vi "orderbook.test.vi"() -> ()   [LabVIEW 2020]
uses:
  orderbook.command.type.ctl
  orderbook.variables.ctl
  application/orderbook.entry.ctl
  application/orderbook.result.type.ctl
  orderbook.state.ctl
  orderbook.memory.states.ctl
  <vilib>/Platform/TimedLoop/XDataNode/timing_clust.ctl
  <vilib>/Platform/TimedLoop/XDataNode/nitl_modes.ctl
  <vilib>/Platform/TimedLoop/XDataNode/wakeup.ctl
  orderbook.command.ctl
  <vilib>/rvi/Emulation/niFpgaSctlEmulationGetInTimedLoop.vi
  <vilib>/rvi/Emulation/niFpgaEmulationReportErrorSimple.vi
  <vilib>/rvi/Emulation/niFpgaGetClockAttributes.vi
  <vilib>/rvi/Emulation/niFpgaCriticalErrorInLSC.vi
  <vilib>/rvi/interface/RandomDataEmulation/nirviRandomDataMultiElementFPGAFIFO.vi
  <instcachedir>/0/nirviRandomDataMultiElementFPGAFIFO_3E9965BA1FAD4E7B8DABA31768A09B1F.lvgen/nirviRandomDataMultiElementFPGAFIFO_3E9965BA1FAD4E7B8DABA31768A09B1F_002.vi
  <vilib>/rvi/interface/RandomDataEmulation/niFpgaRandomDataHandleErrors.vi
  <vilib>/rvi/DataTransferAndStorage/Container/Common/niFpgaContainerExecOnDevCompGetState.vi
  <vilib>/rvi/Emulation/niFpgaEmulationIsFPGAContextNoSignature.vi
  <vilib>/rvi/errors/niFpgaSetErrorForExecOnDevCompSimple.vi
  <vilib>/rvi/eio/common/nirviEmuReportErrorAndStop.vi
  <vilib>/rvi/DataTransferAndStorage/Container/Common/niFpgaContainerGetUniqueNameForEmu.vi
  <vilib>/rvi/FIFO/Fifo_Resource/nirvififoEmulationSetSize.vi
  <vilib>/rvi/FIFO/Fifo_Resource/nirviFifoEmulationQueueMgr.vi
  <instcachedir>/0/nirviFifoEmulationQueueMgr_E5CAEC123FF24DC58D834DCA3CDAA9B5.lvgen/nirviFifoEmulationQueueMgr_E5CAEC123FF24DC58D834DCA3CDAA9B5_018.vi
  <vilib>/rvi/FIFO/Fifo_Resource/nirvififoEmulationDetermineInputValidOut.vi
  <vilib>/rvi/FIFO/Fifo_Resource/nirvififoEmulationCreateLock.vi
  <vilib>/rvi/Emulation/niFpgaProcessEmulError.vi
  <vilib>/rvi/FIFO/Fifo_Resource/nirvififoEmulationObtainLock.vi
  <vilib>/rvi/FIFO/Fifo_Resource/nirvififoEmulationReleaseLock.vi
  <vilib>/rvi/occurrence/nirviWaitOnOccurrenceBase.vi
  <vilib>/rvi/errors/nirviReportUnexpectedCaseInternalError.vi
  <vilib>/rvi/errors/nirviReportUnexpectedCaseInternalError (U32).vi
  <vilib>/Utility/error.llb/Clear Errors.vi
  <instcachedir>/0/nirviFifoEmulationQueueMgr_E5CAEC123FF24DC58D834DCA3CDAA9B5.lvgen/nirviFifoEmulationQueueMgr_E5CAEC123FF24DC58D834DCA3CDAA9B5_017.vi
  <vilib>/Platform/TimedLoop/XDataNode/XDataNode.xnode
  <vilib>/rvi/DataTransferAndStorage/Container/XNode/niFpgaContainer.xnode
  <vilib>/rvi/interface/RandomDataEmulation/nirviRandomDataFpgaMultiElementTemplate.vi
  <vilib>/rvi/FIFO/Fifo_Resource/niFpgaFifoEmulationRefIn.vi
  <vilib>/Platform/TimedLoop/XDataNode/XDNodeRunTimeDep.lvlib
panel:
  out "OrderBook.Variables":T1={"Write.Request"=FALSE, "Read.Request"=FALSE, "Read.Address"=0, "Read.OrderBook.Entry"={"OrderBook Result"=enum."Result.Found", "Side (U8)"=0, "Order Id (U64)"=0, "Quantity (U32)"=0, "Symbol (U64)"=0, "Price (U64)"=0, "Other Metric (U32)"=0, "Other Metric 2 (U32)"=0}, "Number.of.Entries"=0, "OrderBook.State"=enum."Reset", "Ready.For.OrderBook.Command"=FALSE, "Memory.State"=enum."Write", "Move"=FALSE, "Read.Valid"=FALSE, "Write.Address"=0, "Write.OrderBook.Entry"={"OrderBook Result"=enum."Result.Found", "Side (U8)"=0, "Order Id (U64)"=0, "Quantity (U32)"=0, "Symbol (U64)"=0, "Price (U64)"=0, "Other Metric (U32)"=0, "Other Metric 2 (U32)"=0}, "OrderBook.Result.Valid"=FALSE, "AddOrder.Count"=0, "Query.Count"=0, "Reset.Count"=0, "Wait.Count"=0}
  in  "Reset":bool
  in  "OrderBook Command":T6
  in  "Cancelled Quantity (U32)":u32
  in  "Executed Quantity (U32)":u32
  in  "Price (U64)":u64
  in  "Symbol (U64)":u64
  in  "Quantity (U32)":u32
  in  "Order Id (U64)":u64
  in  "Side (U8)":u8
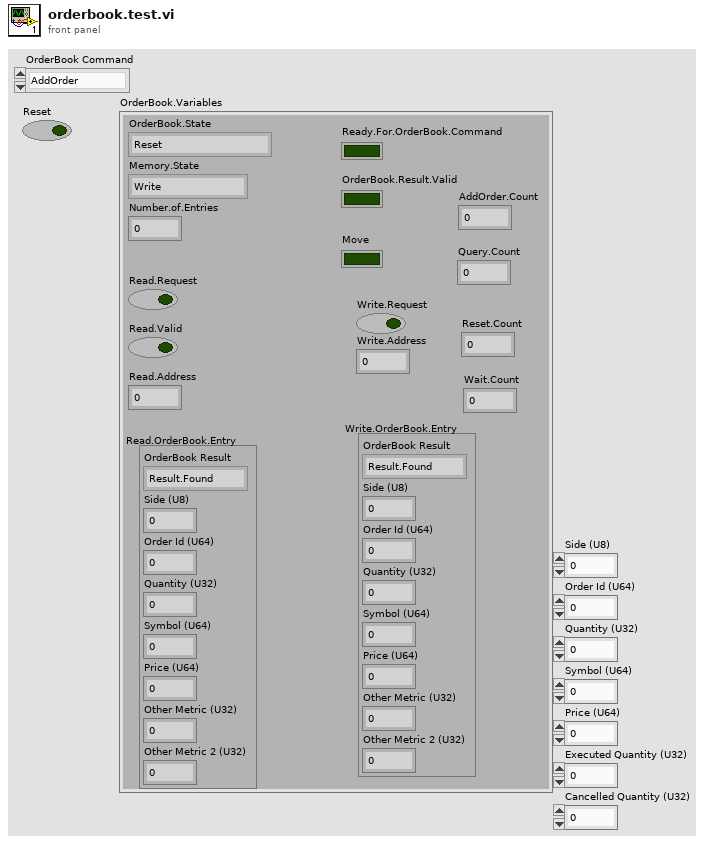
[diagram p1: front panel]
types:
  T1 = typedef "orderbook.variables.ctl" = cluster{"Write.Request":bool, "Read.Request":bool, "Read.Address":u32, "Read.OrderBook.Entry":T2, "Number.of.Entries":u32, "OrderBook.State":T4, "Ready.For.OrderBook.Command":bool, "Memory.State":T5, "Move":bool, "Read.Valid":bool, "Write.Address":u32, "Write.OrderBook.Entry":T2, "OrderBook.Result.Valid":bool, "AddOrder.Count":u32, "Query.Count":u32, "Reset.Count":u32, "Wait.Count":u32}
  T2 = typedef "orderbook.entry.ctl" = cluster{"OrderBook Result":T3, "Side (U8)":u8, "Order Id (U64)":u64, "Quantity (U32)":u32, "Symbol (U64)":u64, "Price (U64)":u64, "Other Metric (U32)":u32, "Other Metric 2 (U32)":u32}
  T3 = typedef "orderbook.result.type.ctl" = enum16{"Result.Found", "Result.Not.Found"}
  T4 = typedef "orderbook.state.ctl" = enum16{"Reset", "WaitForNewCommand", "AddOrder", "Query"}
  T5 = typedef "orderbook.memory.states.ctl" = enum16{"New", "Write", "Request.Data", "Wait.For.Data", "Data.Ready"}
  T6 = typedef "orderbook.command.type.ctl" = enum16{"AddOrder", "OrderExecuted", "ReduceSize", "ModifyOrder", "DeleteOrder", "Query"}
  T7 = typedef "XDNodeRunTimeDep.lvlib/timing_clust.ctl" = cluster{"Expected End [f-1]":u64, "Actual End [f-1]":u64, "Finished Late? [f-1]":bool, "Expected End [i-1]":u64, "Actual End [i-1]":u64, "Finished Late? [i-1]":bool, "Expected Start [i]":u64, "Actual Start [i]":u64, "Expected Start [f]":u64, "Actual Start [f]":u64, "Source Name":string, "Structure Name":string, "Period":i64, "Deadline":i64, "Offset":i64, "Start":i64, "Priority":i32, "Timeout":i32, "Mode":T8, "Wakeup Reason":T9, "Error":errorcluster, "Source Type":string, "Secondary Source Type":string, "Global End Time":u64, "Global Start Time":u64, "Frame Duration":u64, "Iteration Duration":u64, "Assigned CPU":i32, "I/O Scan Engine Mode":u32}
  T8 = typedef "XDNodeRunTimeDep.lvlib/nitl_modes.ctl" = enum32{"No Change", "Process missed periods, maintain original phase", "Discard missed periods, maintain original phase", "Process missed periods, ignore original phase", "Discard missed periods, ignore original phase"}
  T9 = typedef "XDNodeRunTimeDep.lvlib/wakeup.ctl" = enum32{"Normal", "Aborted", "Asynchronous wakeup", "Timing source error", "Timed loop error", "Timeout"}
  T10 = typedef "orderbook.command.ctl" = cluster{"OrderBook Command.Type":T6, "Side (U8)":u8, "Order Id (U64)":u64, "Quantity (U32)":u32, "Symbol (U64)":u64, "Price (U64)":u64, "Executed Quantity (U32)":u32, "Cancelled Quantity (U32)":u32}
  T11 = cluster{"OrderBook Command.Type":enum16{"AddOrder", "OrderExecuted", "ReduceSize", "ModifyOrder", "DeleteOrder", "Query"}, "Side (U8)":u8, "Order Id (U64)":u64, "Quantity (U32)":u32, "Symbol (U64)":u64, "Price (U64)":u64, "Executed Quantity (U32)":u32, "Cancelled Quantity (U32)":u32}
  T12 = cluster{"OrderBook Result":enum16{"Result.Found", "Result.Not.Found"}, "Side (U8)":u8, "Order Id (U64)":u64, "Quantity (U32)":u32, "Symbol (U64)":u64, "Price (U64)":u64, "Other Metric (U32)":u32, "Other Metric 2 (U32)":u32}
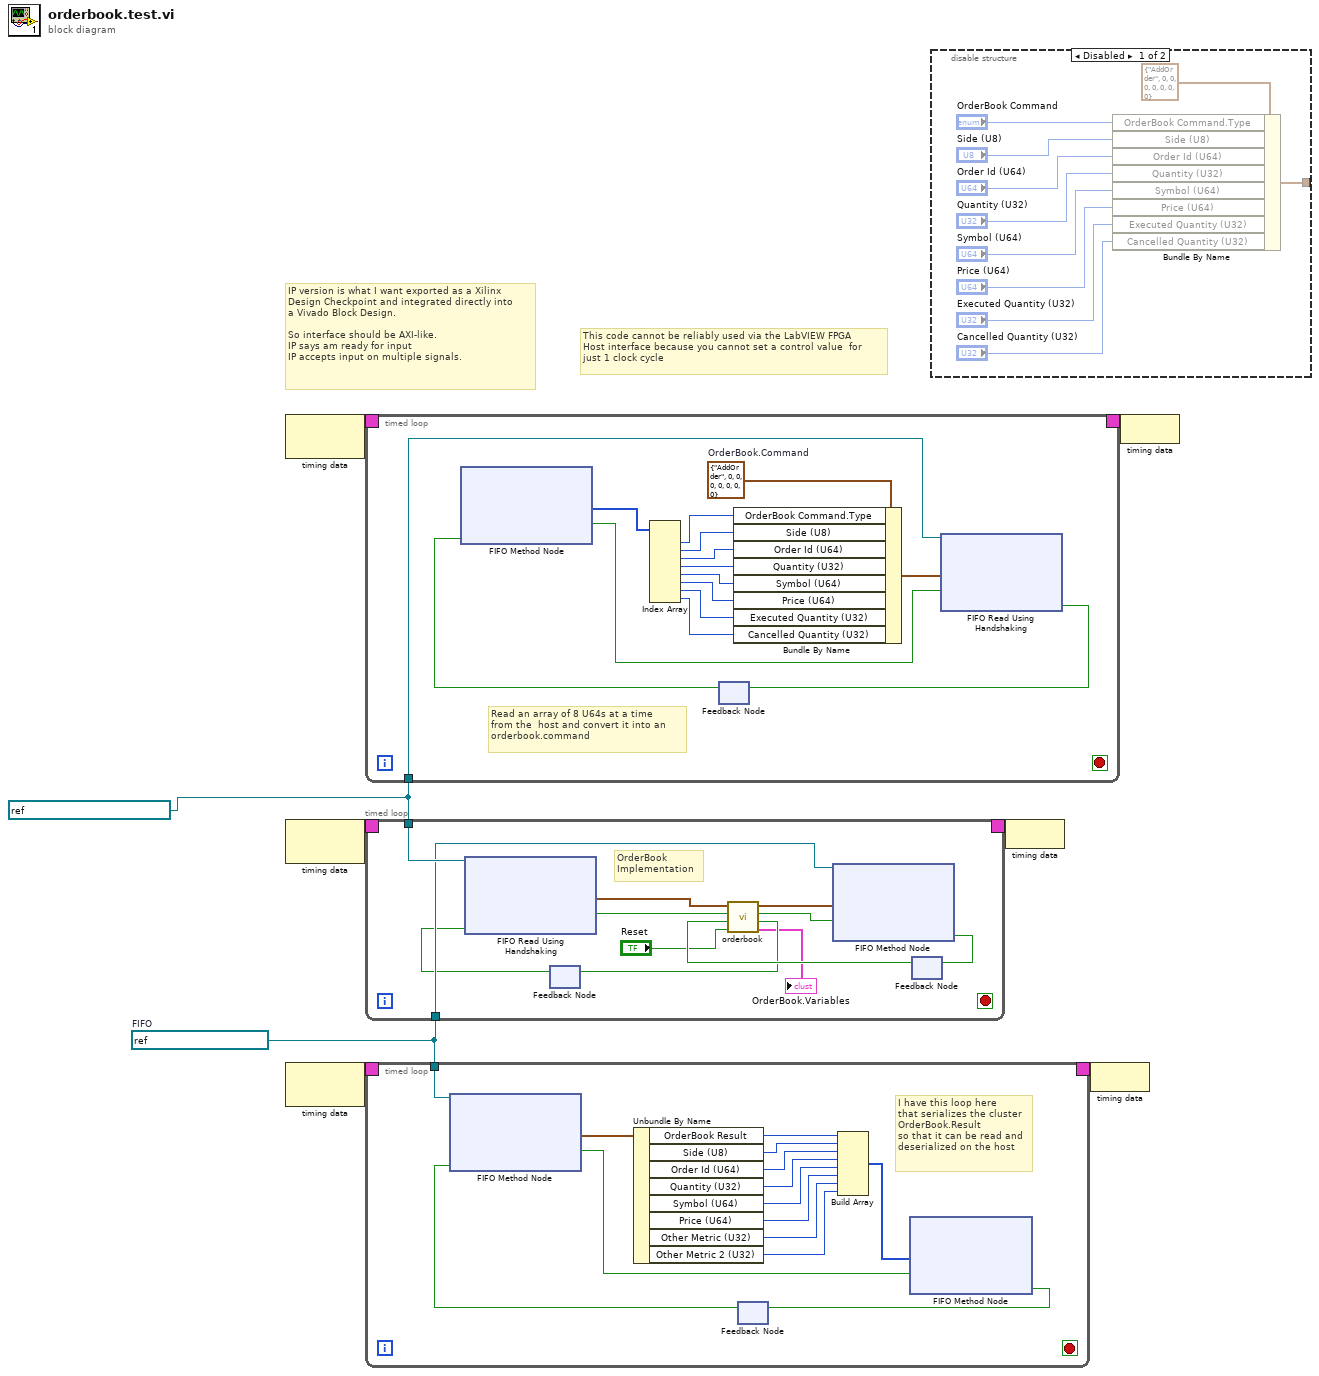
[diagram p0: block diagram]
diagram:
  w1 = refnum<k21> "TS-OrderBook.Command" ("FIFO In")
  w2 = refnum<k21> "TS-OrderBook.Result"  # FIFO
  # "This code cannot be reliably used via the LabVIEW FPGA\nHost interface because you cannot set a control value  for\njust 1 clock cycle"
  # "IP version is what I want exported as a Xilinx\nDesign Checkpoint and integrated directly into\na Vivado Block Design.\n\nSo interface should be AXI-like.\nIP says am ready for input\nIP accepts input on multiple signals."
  n1 = node-c288() -> (w8:T7)  [unwired: 1 in]
  n2 = node-c288() -> (w6:T7)  [unwired: 1 in]
  n3 = node-c288() -> (w4:T7)  [unwired: 1 in]
  n4 = timed-loop {
    timing: w8 -> [_]
    timing-out: [_] -> w7
    tunnel: w1 -> [w23]
    stop <- _ stop-if-true
    w15 = T10 {"OrderBook Command.Type"=enum."AddOrder", "Side (U8)"=0, "Order Id (U64)"=0, "Quantity (U32)"=0, "Symbol (U64)"=0, "Price (U64)"=0, "Executed Quantity (U32)"=0, "Cancelled Quantity (U32)"=0}  # OrderBook.Command
    # "Read an array of 8 U64s at a time\nfrom the  host and convert it into an \norderbook.command"
    n5 = feedback #1() -> (w21:bool)  [unwired: 1 in]
    n6 = xnode ("FIFO Method Node")("Ready for Output"=w21) -> ("Element"=w20:u64[], "Output Valid"=w9:bool)  [unwired: 1 in, 1 out]
    n7 = Index Array(array=w20) -> (element #1=w19:u64, element #2=w18:u64, element #3=w17:u64, element #4=w16:u64, element #5=w13:u64, element #6=w12:u64, element #7=w11:u64, element #8=w10:u64)  [unwired: 8 in]
    n8 = Bundle By Name(cluster=w15, "OrderBook Command.Type"=w19, "Side (U8)"=w18, "Order Id (U64)"=w17, "Quantity (U32)"=w16, "Symbol (U64)"=w13, "Price (U64)"=w12, "Executed Quantity (U32)"=w11, "Cancelled Quantity (U32)"=w10) -> (w14:T10)
    n9 = xnode ("FIFO Read Using Handshaking")("Element"=w14, "Input Valid"=w9, "FIFO In"=w23) -> ("Ready for Input"=w22:bool)  [unwired: 1 out]
    n10 = feedback-in #1(w22) -> ()
  }
  n11 = timed-loop {
    timing: w6 -> [_]
    timing-out: [_] -> w5
    tunnel: w1 -> [w37]
    tunnel: w2 -> [w35]
    stop <- _ stop-if-true
    # "OrderBook\nImplementation"
    n12 = feedback #2() -> (w28:bool)  [unwired: 1 in]
    n13 = xnode ("FIFO Read Using Handshaking")("Ready for Output"=w28, "FIFO In"=w37) -> ("Element"=w34:T11, "Output Valid"=w33:bool)  [unwired: 1 out]
    n14 = feedback #3() -> (w32:bool)  [unwired: 1 in]
    n15 = call "orderbook.vi"("Reset"="Reset", "Ready.For.OrderBook.Result"=w32, "OrderBook.Command.Valid"=w33, "OrderBook.Command"=w34) -> ("OrderBook.Variables"=→"OrderBook.Variables":T1, "Ready.For.OrderBook.Command"=w29:bool, "OrderBook.Result.Valid"=w30:bool, "OrderBook.Entry"=w31:T2)  [unwired: 4 in]
    n16 = feedback-in #2(w29) -> ()
    n17 = xnode ("FIFO Method Node")("Element"=w31, "Input Valid"=w30, "FIFO In"=w35) -> ("Ready for Input"=w36:bool)  [unwired: 1 out]
    n18 = feedback-in #3(w36) -> ()
  }
  n19 = timed-loop {
    timing: w4 -> [_]
    timing-out: [_] -> w3
    tunnel: w2 -> [w53]
    stop <- _ stop-if-true
    # "I have this loop here\nthat serializes the cluster\nOrderBook.Result\nso that it can be read and\ndeserialized on the host"
    n20 = feedback #4() -> (w51:bool)  [unwired: 1 in]
    n21 = xnode ("FIFO Method Node")("Ready for Output"=w51, "FIFO In"=w53) -> ("Element"=w49:T12, "Output Valid"=w50:bool)  [unwired: 1 out]
    n22 = Unbundle By Name(w49) -> ("OrderBook Result"=w48:enum16{"Result.Found", "Result.Not.Found"}, "Side (U8)"=w47:u8, "Order Id (U64)"=w46:u64, "Quantity (U32)"=w45:u32, "Symbol (U64)"=w43:u64, "Price (U64)"=w42:u64, "Other Metric (U32)"=w41:u32, "Other Metric 2 (U32)"=w44:u32)
    n23 = Build Array(w48, w47, w46, w45, w43, w42, w41, w44) -> (w40:u64[])
    n24 = xnode ("FIFO Method Node")("Element"=w40, "Input Valid"=w50) -> ("Ready for Input"=w52:bool)  [unwired: 1 in, 1 out]
    n25 = feedback-in #4(w52) -> ()
  }
  n26 = disable-structure shown="Disabled" {
    disable-tunnel: [w56 _] -> _
    frame Disabled {
      n27 = Bundle By Name(cluster=T10 {"OrderBook Command.Type"=enum."AddOrder", "Side (U8)"=0, "Order Id (U64)"=0, "Quantity (U32)"=0, "Symbol (U64)"=0, "Price (U64)"=0, "Executed Quantity (U32)"=0, "Cancelled Quantity (U32)"=0} ("Cluster"), "OrderBook Command.Type"="OrderBook Command", "Side (U8)"="Side (U8)", "Order Id (U64)"="Order Id (U64)", "Quantity (U32)"="Quantity (U32)", "Symbol (U64)"="Symbol (U64)", "Price (U64)"="Price (U64)", "Executed Quantity (U32)"="Executed Quantity (U32)", "Cancelled Quantity (U32)"="Cancelled Quantity (U32)") -> (w56:T10)
    }
    frame Enabled {
    }
  }
  n28 = node-c288(w5) -> ()
  n29 = node-c288(w3) -> ()
  n30 = node-c288(w7) -> ()
